vi "InitializePIStageOutputChannels.vi"(1 "1st Axis":u16(ring) items=["x", "y"]) -> (0 "Append Channels":tag)   [LabVIEW 2009]
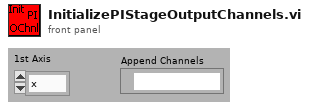
[diagram p1: front panel]
types:
  T1 = typedef "StageSettings.ctt" = cluster{"channels (x, y, z)":tag, "Stage Scaling (V/µm)":dbl}
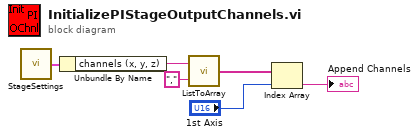
[diagram p0: block diagram]
diagram:
  n1 = call "StageSettings.vi"() -> ("PI Stage Setup (output)"=w6:T1)  [unwired: 2 in]
  n2 = Unbundle By Name(w6) -> ("channels (x, y, z)"=w5:tag)
  n3 = call "ListToArray.vi"("delimiter"=",", "list"=w5) -> ("Array"=w3:string[])
  n4 = Index Array(array=w3, index="1st Axis") -> (element=→"Append Channels":string)
